vi "Write VI Path.vi"(8 "error in (no error)":errorcluster, 10 "VI Path":path, 11 "Run VI in":refnum<class "Run VI.lvclass">) -> (0 "error out":errorcluster, 3 "Run VI out":refnum<class "Run VI.lvclass">)   [LabVIEW 2014, in "Run VI.lvclass"]
uses:
  Run VI.lvclass
  Run VI.lvclass/Run VI.ctl
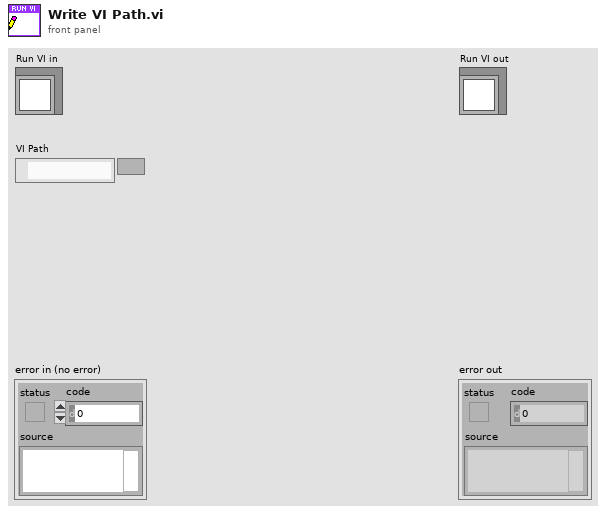
[diagram p1: front panel]
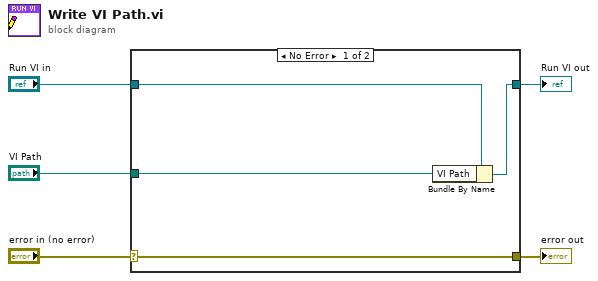
[diagram p0: block diagram]
diagram:
  n1 = case shown="No Error" "error in (no error)" {
    selector: "error in (no error)" -> [w9 w10]
    tunnel: [w9 w10] -> w4
    tunnel: [w7 w11] -> w2
    tunnel: "Run VI in" -> [w8 w11]
    tunnel: "VI Path" -> [w6 _]
    frame No Error {
      n2 = Bundle By Name(cluster=w8, "VI Path"=w6) -> (w7:refnum<class "Run VI.lvclass">)
    }
    frame Error {
    }
  }
  "error out" <- w4
  "Run VI out" <- w2
